vi "remap tag and channel.vi"(8 "error in":errorcluster, 9 "tag name":string, 10 "channel":refnum<class "TBM channel.lvclass">, 11 "engine configuration in":refnum<class "engine configuration.lvclass">) -> (0 "error out":errorcluster, 3 "engine configuration out":refnum<class "engine configuration.lvclass">)   [LabVIEW 2013, in "user tag bus module editor node.lvclass"]
uses:
  user tag bus module editor node.lvclass
  <vilib>/NI/Module Execution Interface/Engine Configuration/engine configuration.lvclass
  <vilib>/NI/Tag Bus Module Framework/channel/TBM channel.lvclass
  <vilib>/NI/Configuration Framework/serializable configuration/NISE_CEF_serializable configuration.lvclass/NISE_CEF_serializable configuration.ctl
  <vilib>/NI/Configuration Framework/serializable configuration/NISE_CEF_serializable configuration.lvclass
  <vilib>/NI/Tag Bus/tag/tag descriptor.lvclass/tag descriptor.ctl
  <vilib>/NI/Tag Bus/tag/write tag name.vi
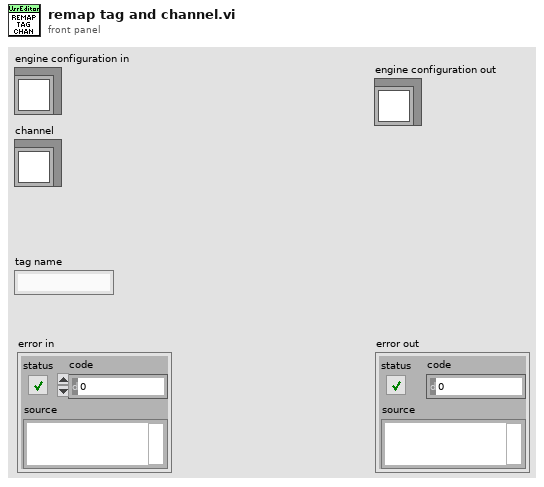
[diagram p1: front panel]
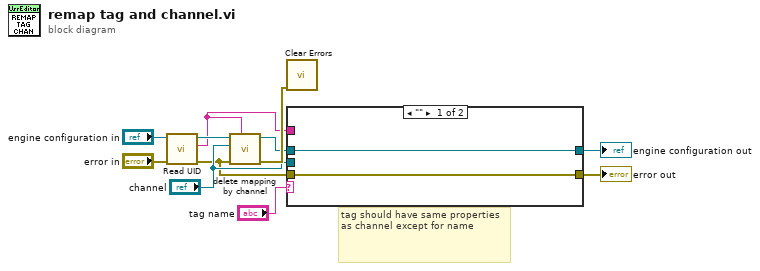
[diagram p0: block diagram]
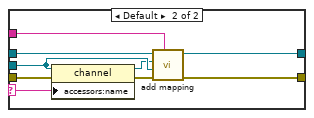
[diagram p2: hidden frame]
diagram:
  # "tag should have same properties as channel except for name"
  n1 = call <vilib>:"Read UID.vi"("error in"="error in", "configuration in"="engine configuration in") -> ("error out"=w4:errorcluster, "instance id"=w1:string, "configuration out"=w2:refnum<class "engine configuration.lvclass">)  [unwired: 7 in]
  n2 = call <vilib>:"delete mapping by channel.vi"("owner ID"=w1, "error in"=w4, "channel"="channel", "engine configuration in"=w2) -> ("error out"=w11:errorcluster, "engine configuration out"=w6:refnum<class "engine configuration.lvclass">)  [unwired: 6 in]
  n3 = call <vilib>:"Clear Errors.vi"("error in (no error)"=w11) -> ()  [unwired: 6 in, 1 out]
  n4 = case shown="\"\"" "tag name" {
    selector: "tag name" -> [_ w14]
    tunnel: w4 -> [w12 w22]
    tunnel: w1 -> [_ w21]
    tunnel: [w12 w20] -> w9
    tunnel: [w13 w19] -> w8
    tunnel: "channel" -> [_ w17]
    tunnel: w6 -> [w13 w15]
    frame "" {
    }
    frame Default {
      n5 = property class="channel"(reference=w17, error in=w22, "accessors:name"=w14) -> (reference out=w16:refnum<class "TBM channel.lvclass">, error out=w18:errorcluster)
      n6 = call <vilib>:"add mapping.vi"("owner ID"=w21, "error in"=w18, "channel"=w17, "tag descriptor"=w16, "engine configuration"=w15) -> ("error out"=w20:errorcluster, "engine configuration out"=w19:refnum<class "engine configuration.lvclass">)  [unwired: 5 in]
    }
  }
  "error out" <- w9
  "engine configuration out" <- w8
